vi "circuits-resistor-2.vi"(1 "Invert Y":bool, 2 "Invert X":bool, 4 "L3":dbl=2.0, 5 "L2":dbl=1.0, 6 "Swap-XY":bool, 7 "L1":dbl=1.0, 8 "Device in Y":refnum<k24>, 9 "GetPOS Y":refnum<vi>, 10 "GetPOS X":refnum<vi>, 11 "Device in X":refnum<k24>) -> (0 "Device out Y":refnum<k24>, 3 "Device out X":refnum<k24>)   [LabVIEW 2014]
doc: "André Romero - 2019\nandretec@ifsc.usp.br"
uses:
  motorsGlobalVar.vi
  C:/user-Lab/AndreTec/GITs/andretec/Thorlabs-Vector-Move/kinesisTec/Kinesis/Thorlabs.MotionControl.TCube.DCServoCLI.dll
  kinesisTec/Kinesis/Thorlabs.MotionControl.TCube.DCServoCLI.dll
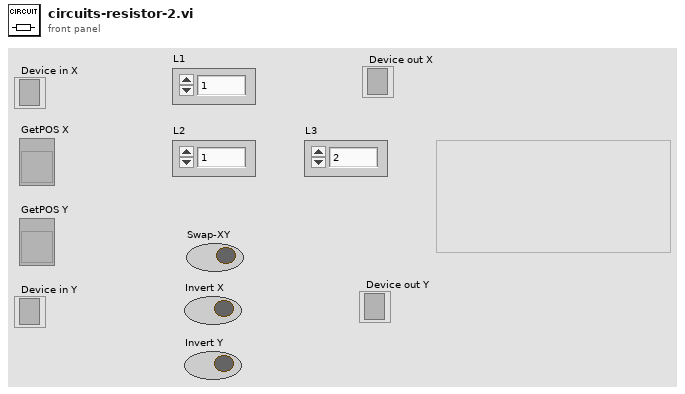
[diagram p1: front panel]
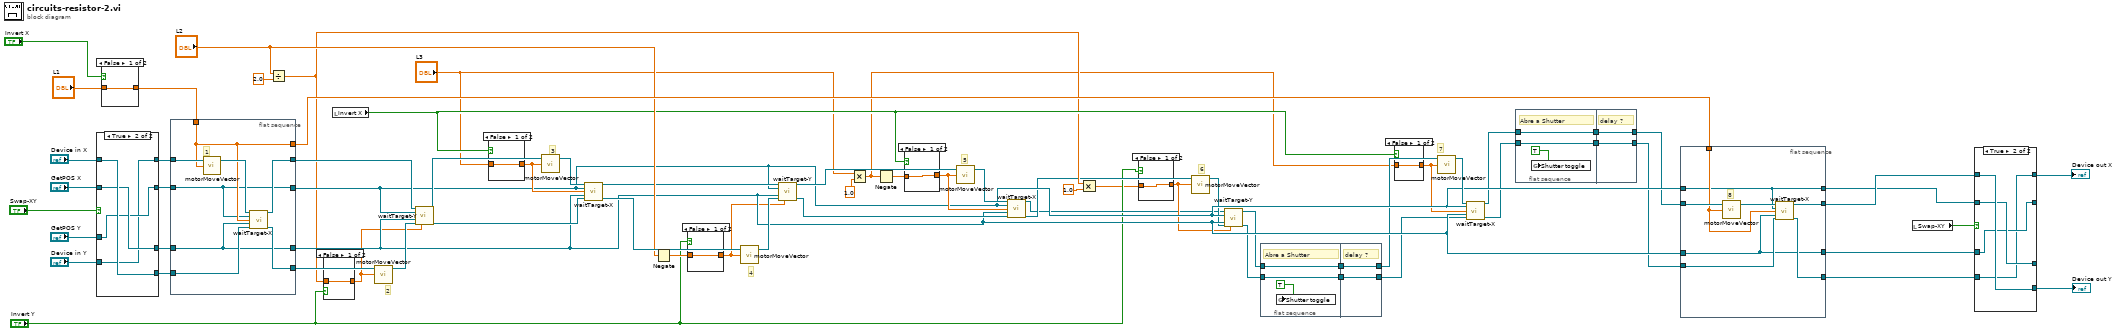
[diagram p0: block diagram]
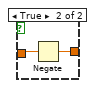
[diagram p3: hidden frame]
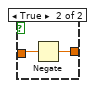
[diagram p4: hidden frame]
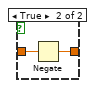
[diagram p5: hidden frame]
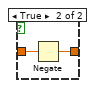
[diagram p6: hidden frame]
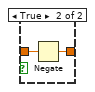
[diagram p7: hidden frame]
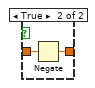
[diagram p8: hidden frame]
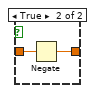
[diagram p9: hidden frame]
diagram:
  # "7"
  # "6"
  # "5"
  # "4"
  # "3"
  # "2"
  n1 = case shown="True" "Swap-XY" {
    tunnel: "Device in X" -> [w70 w76]
    tunnel: [w70 w73] -> w62
    tunnel: "GetPOS Y" -> [w72 w74]
    tunnel: [w72 w75] -> w60
    tunnel: "Device in Y" -> [w71 w73]
    tunnel: [w71 w76] -> w58
    tunnel: "GetPOS X" -> [w69 w75]
    tunnel: [w69 w74] -> w56
    frame False {
    }
    frame True {
    }
  }
  n2 = case shown="False" "Invert X" {
    tunnel: "L1" -> [w77 w79]
    tunnel: [w77 w78] -> w53
    frame False {
    }
    frame True {
      n3 = Negate(x=w79) -> (-x=w78:dbl)
    }
  }
  n4 = flat-sequence {
    tunnel: w62 -> [w87]
    tunnel: [w84] -> w51
    tunnel: w58 -> [w85]
    tunnel: [w83] -> w67
    tunnel: [w81] -> w36
    tunnel: [w80] -> w35
    tunnel: [w82] -> w68
    tunnel: w53 -> [w82]
    tunnel: w56 -> [w81]
    tunnel: w60 -> [w80]
    frame #0 {
      # "1"
      n5 = call "motorMoveVector.vi"("Distance"=w82, "Device in"=w87) -> ("Device out"=w86:refnum<k24>)  [unwired: 3 in]
      n6 = call "waitTarget-X.vi"("Device in X"=w86, "GetPOS X"=w81, "Position X"=w82, "GetPOS Y"=w80, "Device in Y"=w85) -> ("Device out X"=w84:refnum<k24>, "Device out Y"=w83:refnum<k24>)  [unwired: 7 in, 2 out]
    }
  }
  n7 = Divide(x="L2", y=2.0) -> (x/y=w31:dbl)
  n8 = case shown="False" "Invert Y" {
    tunnel: w31 -> [w88 w90]
    tunnel: [w88 w89] -> w34
    frame False {
    }
    frame True {
      n9 = Negate(x=w90) -> (-x=w89:dbl)
    }
  }
  n10 = local read "Invert X"() -> (w37:bool)
  n11 = call "motorMoveVector.vi"("Distance"=w34, "Device in"=w67) -> ("Device out"=w66:refnum<k24>)  [unwired: 3 in]
  n12 = call "waitTarget-Y.vi"("Device in X"=w51, "GetPOS X"=w36, "GetPOS Y"=w35, "Device in Y"=w66, "Position Y"=w34) -> ("Device out X"=w50:refnum<k24>, "Device out Y"=w48:refnum<k24>)  [unwired: 7 in, 2 out]
  n13 = case shown="False" w37 {
    tunnel: [w91 w92] -> w47
    tunnel: "L3" -> [w91 w93]
    frame False {
    }
    frame True {
      n14 = Negate(x=w93) -> (-x=w92:dbl)
    }
  }
  n15 = call "motorMoveVector.vi"("Distance"=w47, "Device in"=w50) -> ("Device out"=w49:refnum<k24>)  [unwired: 3 in]
  n16 = call "waitTarget-X.vi"("Device in X"=w49, "GetPOS X"=w36, "Position X"=w47, "GetPOS Y"=w35, "Device in Y"=w48) -> ("Device out X"=w43:refnum<k24>, "Device out Y"=w46:refnum<k24>)  [unwired: 7 in, 2 out]
  n17 = Negate(x="L2") -> (-x=w32:dbl)
  n18 = case shown="False" "Invert Y" {
    tunnel: [w94 w95] -> w33
    tunnel: w32 -> [w94 w96]
    frame False {
    }
    frame True {
      n19 = Negate(x=w96) -> (-x=w95:dbl)
    }
  }
  n20 = call "motorMoveVector.vi"("Distance"=w33, "Device in"=w46) -> ("Device out"=w44:refnum<k24>)  [unwired: 3 in]
  n21 = call "waitTarget-Y.vi"("Device in X"=w43, "GetPOS X"=w36, "GetPOS Y"=w35, "Device in Y"=w44, "Position Y"=w33) -> ("Device out X"=w42:refnum<k24>, "Device out Y"=w38:refnum<k24>)  [unwired: 7 in, 2 out]
  n22 = Multiply(x="L3", y=1.0) -> (x*y=w10:dbl)
  n23 = Negate(x=w10) -> (-x=w41:dbl)
  n24 = case shown="False" w37 {
    tunnel: [w97 w98] -> w39
    tunnel: w41 -> [w97 w99]
    frame False {
    }
    frame True {
      n25 = Negate(x=w99) -> (-x=w98:dbl)
    }
  }
  n26 = call "motorMoveVector.vi"("Distance"=w39, "Device in"=w42) -> ("Device out"=w40:refnum<k24>)  [unwired: 3 in]
  n27 = call "waitTarget-X.vi"("Device in X"=w40, "GetPOS X"=w36, "Position X"=w39, "GetPOS Y"=w35, "Device in Y"=w38) -> ("Device out X"=w26:refnum<k24>, "Device out Y"=w28:refnum<k24>)  [unwired: 7 in, 2 out]
  n28 = Multiply(x=w31, y=1.0) -> (x*y=w9:dbl)
  n29 = case shown="False" "Invert Y" {
    tunnel: [w100 w101] -> w30
    tunnel: w9 -> [w100 w102]
    frame False {
    }
    frame True {
      n30 = Negate(x=w102) -> (-x=w101:dbl)
    }
  }
  n31 = call "motorMoveVector.vi"("Distance"=w30, "Device in"=w28) -> ("Device out"=w27:refnum<k24>)  [unwired: 3 in]
  n32 = call "waitTarget-Y.vi"("Device in X"=w26, "GetPOS X"=w36, "GetPOS Y"=w35, "Device in Y"=w27, "Position Y"=w30) -> ("Device out X"=w23:refnum<k24>, "Device out Y"=w21:refnum<k24>)  [unwired: 7 in, 2 out]
  n33 = flat-sequence {
    tunnel: w23 -> [w105]
    tunnel: w21 -> [w104]
    tunnel: [w105] -> w25
    tunnel: [w104] -> w24
    tunnel: [w106] -> w20
    tunnel: [w107] -> w22
    tunnel: w25 -> [w107]
    tunnel: w24 -> [w106]
    frame #0 {
      # "Abre a Shutter"
      n34 = global write "motorsGlobalVar.vi" "Shutter toggle"(TRUE ("Shutter toggle")) -> ()
    }
    frame #1 {
      # "delay ?"
    }
  }
  n35 = case shown="False" w37 {
    tunnel: [w108 w109] -> w29
    tunnel: w10 -> [w108 w110]
    frame False {
    }
    frame True {
      n36 = Negate(x=w110) -> (-x=w109:dbl)
    }
  }
  n37 = call "motorMoveVector.vi"("Distance"=w29, "Device in"=w22) -> ("Device out"=w64:refnum<k24>)  [unwired: 3 in]
  n38 = call "waitTarget-X.vi"("Device in X"=w64, "GetPOS X"=w36, "Position X"=w29, "GetPOS Y"=w35, "Device in Y"=w20) -> ("Device out X"=w17:refnum<k24>, "Device out Y"=w15:refnum<k24>)  [unwired: 7 in, 2 out]
  n39 = flat-sequence {
    tunnel: w17 -> [w113]
    tunnel: w15 -> [w112]
    tunnel: [w113] -> w19
    tunnel: [w112] -> w18
    tunnel: [w114] -> w14
    tunnel: [w115] -> w16
    tunnel: w19 -> [w115]
    tunnel: w18 -> [w114]
    frame #0 {
      # "Abre a Shutter"
      n40 = global write "motorsGlobalVar.vi" "Shutter toggle"(TRUE ("Shutter toggle")) -> ()
    }
    frame #1 {
      # "delay ?"
    }
  }
  n41 = flat-sequence {
    tunnel: w16 -> [w123]
    tunnel: w14 -> [w119]
    tunnel: [w118] -> w5
    tunnel: w35 -> [w117]
    tunnel: w68 -> [w121]
    tunnel: [w120] -> w6
    tunnel: w36 -> [w116]
    tunnel: [w117] -> w4
    tunnel: [w116] -> w3
    frame #0 {
      # "8"
      n42 = call "motorMoveVector.vi"("Distance"=w121, "Device in"=w123) -> ("Device out"=w122:refnum<k24>)  [unwired: 3 in]
      n43 = call "waitTarget-X.vi"("Device in X"=w122, "GetPOS X"=w116, "Position X"=w121, "GetPOS Y"=w117, "Device in Y"=w119) -> ("Device out X"=w120:refnum<k24>, "Device out Y"=w118:refnum<k24>)  [unwired: 7 in, 2 out]
    }
  }
  n44 = local read "Swap-XY"() -> (w7:bool)
  n45 = case shown="True" w7 {
    tunnel: w6 -> [w125 w131]
    tunnel: [w125 w128] -> w2
    tunnel: w4 -> [w127 w129]
    tunnel: [w127 w130] -> _
    tunnel: w5 -> [w126 w128]
    tunnel: [w126 w131] -> w1
    tunnel: w3 -> [w124 w130]
    tunnel: [w124 w129] -> _
    frame False {
    }
    frame True {
    }
  }
  "Device out X" <- w2
  "Device out Y" <- w1
